vi "Read AQS DATA.vi"(8 "error in (no error)":errorcluster, 11 "NMR in":refnum<class "NMR.lvclass">) -> (0 "error out":errorcluster, 1 "Imag Data":i32[](array[numeric]) format="%.0x", 2 "Real Data":i32[](array[numeric]) format="%.0x", 3 "NMR out":refnum<class "NMR.lvclass">, 4 "Transfer time":u32)   [LabVIEW 2011, in "NMR.lvclass"]
uses:
  NMR.lvclass
  NMR.lvclass/NMR.ctl
panel:
  out "unsigned byte array":u8[][](array[numeric]) format="%.0x"
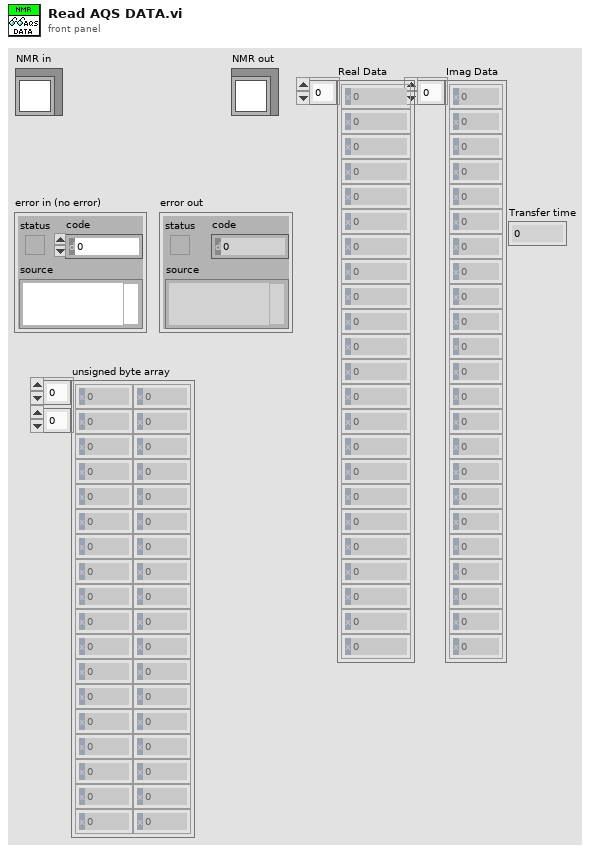
[diagram p1: front panel]
types:
  T1 = typedef "NMR.lvclass/Communication Channel.ctl" = enum16{"VISA", "DLL"}
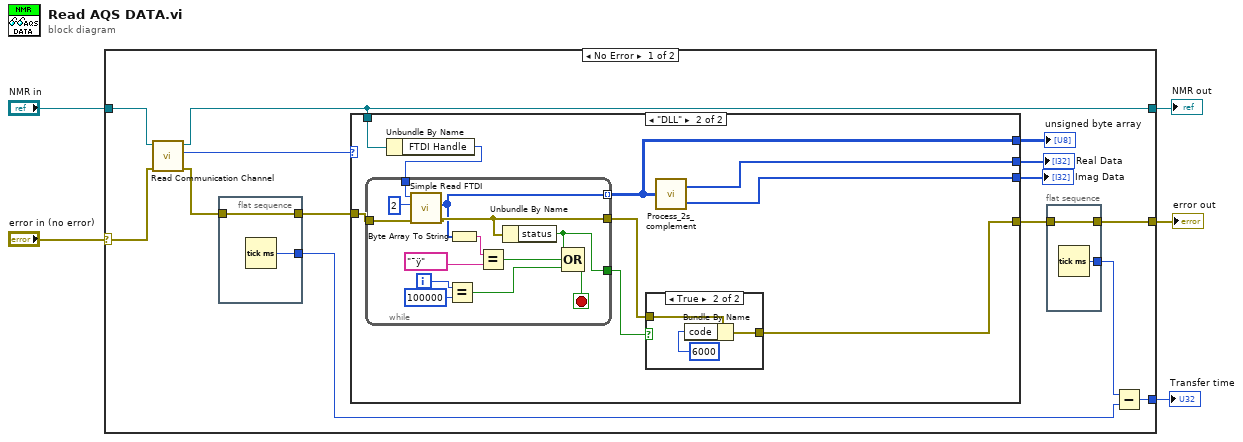
[diagram p0: block diagram]
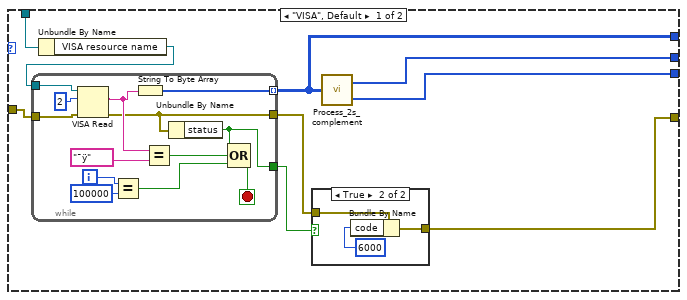
[diagram p2: hidden frame]
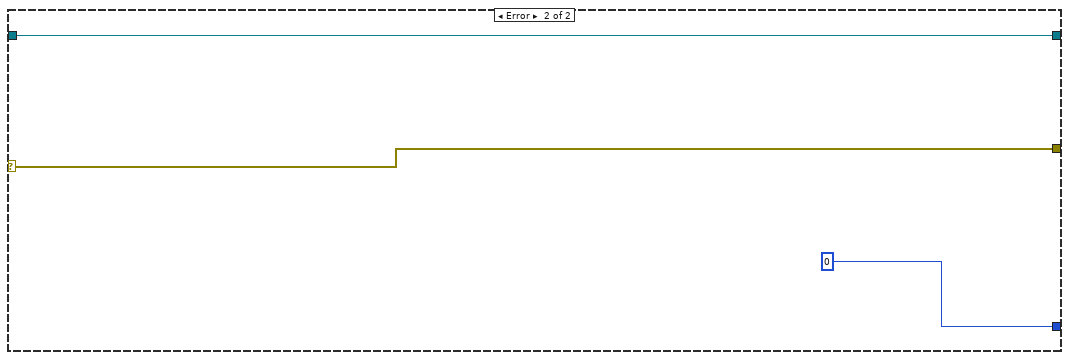
[diagram p5: hidden frame]
diagram:
  n1 = case shown="No Error" "error in (no error)" {
    selector: "error in (no error)" -> [w17 w78]
    tunnel: [w13 w78] -> w4
    tunnel: [w6 w77] -> w2
    tunnel: "NMR in" -> [w18 w77]
    tunnel: [w10 u32 0] -> w1
    frame No Error {
      n2 = call-dynamic "Read Communication Channel.vi"("error in (no error)"=w17, "NMR in"=w18) -> ("error out"=w16:errorcluster, "Communication Channel"=w19:T1, "NMR out"=w6:refnum<class "NMR.lvclass">)  [unwired: 7 in]
      n3 = flat-sequence {
        tunnel: [w23] -> w15
        tunnel: w16 -> [w23]
        tunnel: [w22] -> w11
        frame #0 {
          n4 = Tick Count (ms)() -> (millisecond timer value=w22:u32)
        }
      }
      n5 = case shown="\"DLL\"" w19 {
        tunnel: w15 -> [w32 w51]
        tunnel: [w29 w53] -> w14
        tunnel: [w28 w55] -> w9
        tunnel: [w27 w54] -> w8
        tunnel: [w26 w56] -> w7
        tunnel: w6 -> [w25 w52]
        frame "VISA", Default {
          n6 = Unbundle By Name(w25) -> ("VISA resource name"=w24:refnum<visa-resource-name>)
          n7 = while {
            tunnel: [w49] -> w26 mode=indexing
            tunnel: [w40] -> w30
            tunnel: w24 -> [w39]
            tunnel: w32 -> [w38]
            tunnel: [w37] -> w31
            i -> [w46]
            stop <- w42 stop-if-true
            n8 = VISA Read(VISA resource name=w39, byte count=u32 2, error in (no error)=w38) -> (read buffer=w41:string, error out=w40:errorcluster)  [unwired: 2 out]
            n9 = Equal?(x=w46, y=100000) -> (x = y?=w43:bool)
            n10 = String To Byte Array(string=w41) -> (unsigned byte array=w49:u8[])
            n11 = Equal?(x=w41, y="¯ÿ" ("search string/char (-)")) -> (x = y?=w44:bool)
            n12 = Unbundle By Name(w40) -> ("status"=w37:bool)
            n13 = Compound Arithmetic op=OR(w37, w44, w43) -> (w42:bool)
          }
          n14 = case shown="True" w31 {
            tunnel: w30 -> [w33 w36]
            tunnel: [w33 w35] -> w29
            frame False {
            }
            frame True {
              n15 = Bundle By Name(cluster=w36, "code"=6000 ("y")) -> (w35:errorcluster)
            }
          }
          n16 = call "Process_2s_complement.vi"("uC Raw data"=w26) -> ("Real Data"=w28:i32[], "Imag Data"=w27:i32[])
        }
        frame "DLL" {
          n17 = Unbundle By Name(w52) -> ("FTDI Handle"=w50:u32)
          n18 = while {
            tunnel: [w63] -> w56 mode=indexing
            tunnel: [w65] -> w57
            tunnel: w51 -> [w68]
            tunnel: [w69] -> w58
            tunnel: w50 -> [w66]
            i -> [w74]
            stop <- w70 stop-if-true
            n19 = call "Simple Read FTDI.vi"("error In"=w68, "Bytes To Read"=u32 2 ("byte count"), "FTDI Handle In"=w66) -> ("error out"=w65:errorcluster, "Read Data"=w63:u8[])  [unwired: 6 in, 1 out]
            n20 = Equal?(x=w74, y=100000) -> (x = y?=w71:bool)
            n21 = Byte Array To String(unsigned byte array=w63) -> (string=w64:string)
            n22 = Equal?(x=w64, y="¯ÿ" ("search string/char (-)")) -> (x = y?=w72:bool)
            n23 = Unbundle By Name(w65) -> ("status"=w69:bool)
            n24 = Compound Arithmetic op=OR(w69, w72, w71) -> (w70:bool)
          }
          n25 = case shown="True" w58 {
            tunnel: w57 -> [w59 w62]
            tunnel: [w59 w61] -> w53
            frame False {
            }
            frame True {
              n26 = Bundle By Name(cluster=w62, "code"=6000 ("y")) -> (w61:errorcluster)
            }
          }
          n27 = call "Process_2s_complement.vi"("uC Raw data"=w56) -> ("Real Data"=w55:i32[], "Imag Data"=w54:i32[])
        }
      }
      "Real Data" <- w9
      "Imag Data" <- w8
      "unsigned byte array" <- w7
      n28 = flat-sequence {
        tunnel: [w21] -> w13
        tunnel: w14 -> [w21]
        tunnel: [w20] -> w12
        frame #0 {
          n29 = Tick Count (ms)() -> (millisecond timer value=w20:u32)
        }
      }
      n30 = Subtract(x=w12, y=w11) -> (x-y=w10:u32)
    }
    frame Error {
    }
  }
  "error out" <- w4
  "NMR out" <- w2
  "Transfer time" <- w1
